vi "Process-error.vi"(8 "error in (no error)":errorcluster, 11 "Data in":T1) -> (0 "error out":errorcluster, 3 "Data out":T1)   [LabVIEW 2013, in "MaterialCharacterization.lvlib" / "MC-Main.lvclass"]
uses:
  MC-Main.lvclass
  Object-reference.ctl
  <vilib>/Utility/error.llb/DialogType.ctl
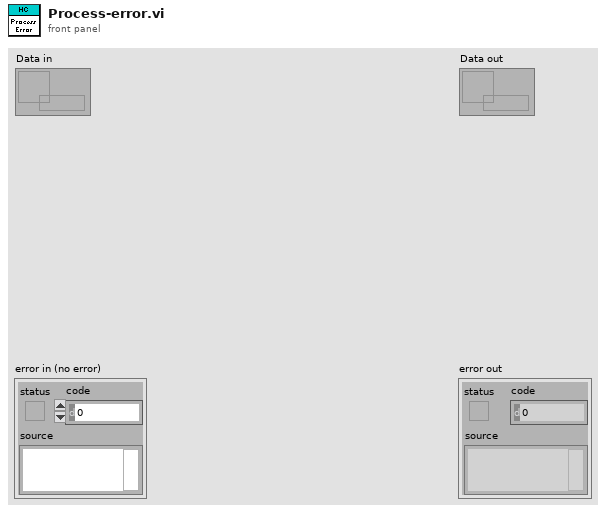
[diagram p1: front panel]
types:
  T1 = typedef "MaterialCharacterization.lvlib/MC-Main.lvclass/Object-reference.ctl" = refnum<data-value>
  T2 = typedef "DialogType.ctl" = u16
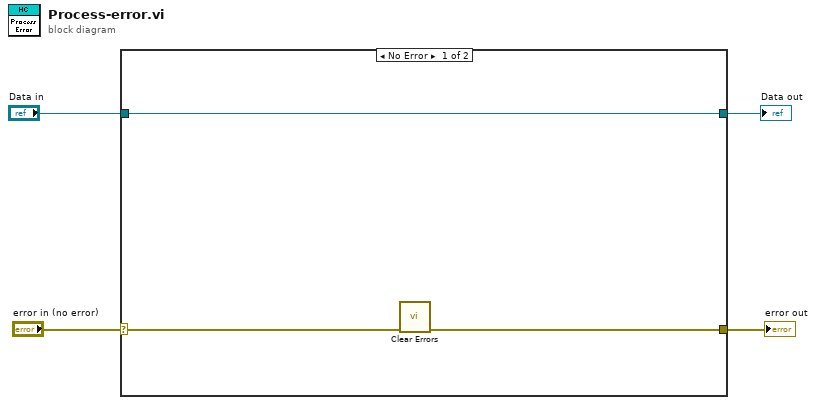
[diagram p0: block diagram]
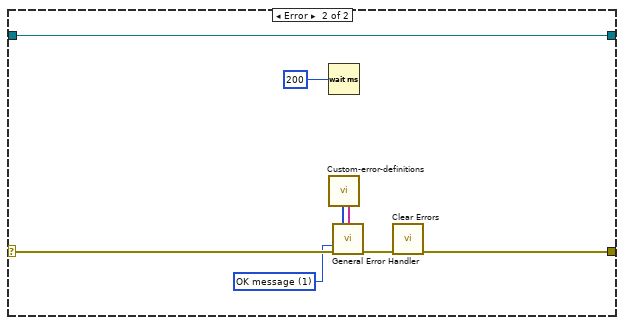
[diagram p2: hidden frame]
diagram:
  n1 = case shown="No Error" "error in (no error)" {
    selector: "error in (no error)" -> [w7 w15]
    tunnel: [w5 w12] -> w3
    tunnel: [w6 w14] -> w1
    tunnel: "Data in" -> [w6 w14]
    frame No Error {
      n2 = call <vilib>:"Clear Errors.vi"("error in (no error)"=w7) -> ("error out"=w5:errorcluster)  [unwired: 6 in]
    }
    frame Error {
      w11 = T2 1 items=["no dialog", "OK message", "continue or stop message", "OK message + warnings", "continue/stop + warnings"] ("type of dialog (OK msg:1)")
      n3 = Wait (ms)(milliseconds to wait=u32 200) -> ()  [unwired: 1 out]
      n4 = call "Custom-error-definitions.vi"() -> ("Descriptions"=w9:string[], "Error codes"=w8:i32[])  [unwired: 9 in, 1 out]
      n5 = call <vilib>:"General Error Handler.vi"("[user-defined codes]"=w8, "[user-defined descriptions]"=w9, "type of dialog (OK msg:1)"=w11, "error in (no error)"=w15) -> ("error out"=w13:errorcluster)  [unwired: 7 in, 4 out]
      n6 = call <vilib>:"Clear Errors.vi"("error in (no error)"=w13) -> ("error out"=w12:errorcluster)  [unwired: 6 in]
    }
  }
  "error out" <- w3
  "Data out" <- w1
